vi "Actor Core.vi"(8 "error in":errorcluster, 11 "Nested in":refnum<class "Productos.lvclass">) -> (0 "error out":errorcluster, 3 "Actor out":refnum<class "Actor.lvclass">)   [LabVIEW 2020, in "Productos.lvlib" / "Productos.lvclass"]
doc: "(<B>Filename</B>: Actor Framework.lvlib:Actor.lvclass:Actor Core.vi)\n\nReceives messages to the actor, reacts to them, and initiates any error handling that may shut the actor down.\n\nDescendant classes may override this VI to append parallel tasks for the actor to complete while it handles messages. Overrides use the Call Parent Method node."
uses:
  Productos.lvclass
  <vilib>/ActorFramework/Actor/Actor.lvclass
  <vilib>/ActorFramework/Stop Msg/Stop Msg.lvclass
  Productos Messages/Producto extraccion Msg/Producto extraccion Msg.lvclass
  Productos Messages/Inventory Msg/Inventory Msg.lvclass
  Productos Messages/Cobro Prod Msg/Cobro Prod Msg.lvclass
panel:
  in  "Cancel Button":bool
  in  "Inventario":bool
  in  "Listo":bool
  out "Total":dbl format="$ %#_6f"
  in  "Chicles":bool
  in  "Cacahuates":bool
  in  "Galletas":bool
  in  "Chocolate":bool
  in  "Sabritas":bool
  in  "Doritos":bool
  in  "Pepsi":bool
  in  "Coca":bool
  out "Productos":T1
  # "Para realizar su pedido haga click en el boton de lo que vaya a ordenar"
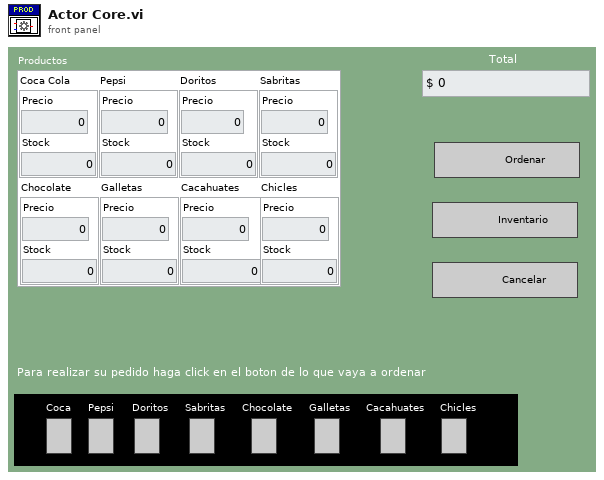
[diagram p1: front panel]
types:
  T1 = cluster{"Coca Cola":cluster{"Precio":dbl, "Stock":dbl}, "Pepsi":cluster{"Precio":dbl, "Stock":dbl}, "Doritos":cluster{"Precio":dbl, "Stock":dbl}, "Sabritas":cluster{"Precio":dbl, "Stock":dbl}, "Chocolate":cluster{"Precio":dbl, "Stock":dbl}, "Galletas":cluster{"Precio":dbl, "Stock":dbl}, "Cacahuates":cluster{"Precio":dbl, "Stock":dbl}, "Chicles":cluster{"Precio":dbl, "Stock":dbl}}
  T2 = cluster{"Stop":refnum<user-event>, "Total":refnum<user-event>, "Productos":refnum<user-event>}
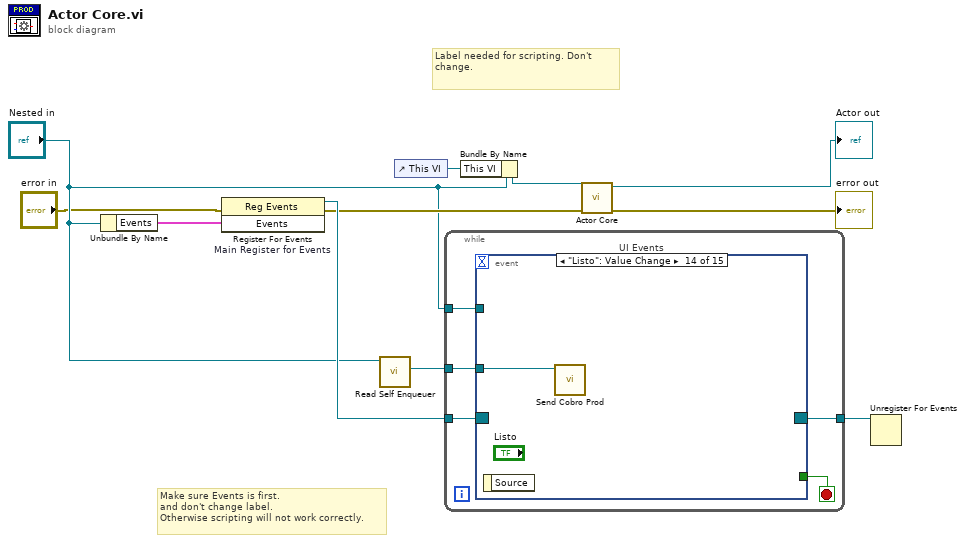
[diagram p0: block diagram]
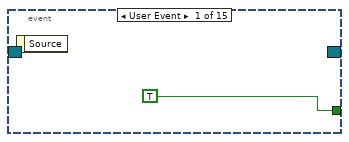
[diagram p2: hidden frame]
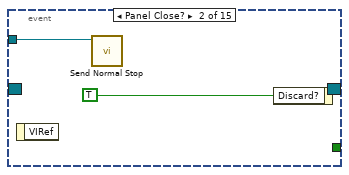
[diagram p3: hidden frame]
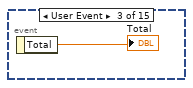
[diagram p4: hidden frame]
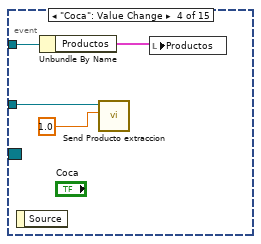
[diagram p5: hidden frame]
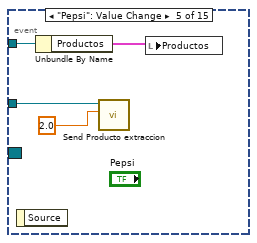
[diagram p6: hidden frame]
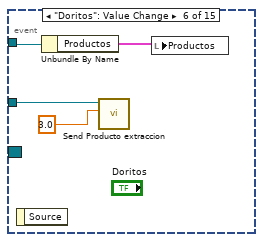
[diagram p7: hidden frame]
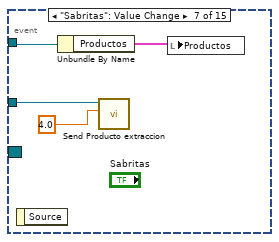
[diagram p8: hidden frame]
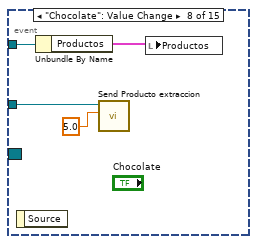
[diagram p9: hidden frame]
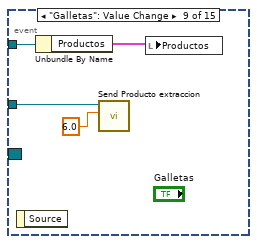
[diagram p10: hidden frame]
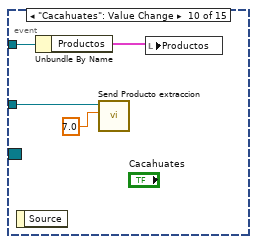
[diagram p11: hidden frame]
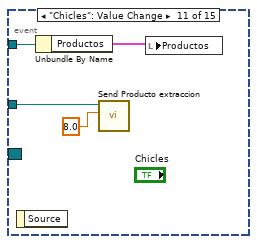
[diagram p12: hidden frame]
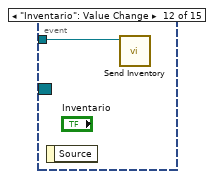
[diagram p13: hidden frame]
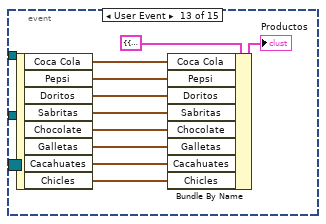
[diagram p14: hidden frame]
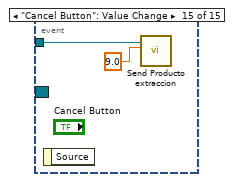
[diagram p15: hidden frame]
diagram:
  # "Label needed for scripting. Don't change."
  # "Make sure Events is first.\nand don't change label.\nOtherwise scripting will not work correctly."
  n1 = Unbundle By Name("Nested in") -> ("Events"=w8:T2)
  n2 = register-events "Main Register for Events"(error in="error in", w8) -> (reference out=w9:refnum<event-registration>, error out=w5:errorcluster)  [unwired: 1 in]
  n3 = call <vilib>:"Read Self Enqueuer.vi"("Actor"="Nested in") -> ("Self Enqueuer"=w6:refnum<class "Message Enqueuer.lvclass">)  [unwired: 10 in]
  n4 = control-ref of="This VI"() -> (w3:refnum<vi>)
  n5 = while {
    tunnel: w9 -> [w16]
    tunnel: [w14] -> w7
    tunnel: w6 -> [w13]
    tunnel: "Nested in" -> [w12]
    stop <- w15 stop-if-true
    n6 = event "UI Events" shown="[13] \"Listo\": Value Change" {
      selector: w16 -> [_ _ _ _ _ _ _ _ _ _ _ _ _ _ _]
      dyn-events: [_ _ _ _ _ _ _ _ _ _ _ _ _ _ _] -> w14
      timeout: _ -> [_ _ _ _ _ _ _ _ _ _ _ _ _ _ _]
      tunnel: [TRUE _ _ _ _ _ _ _ _ _ _ _ _ _ _] -> w15
      tunnel: w13 -> [_ w18 _ w24 w28 w32 w36 w40 w44 w48 w52 w53 _ w64 w65]
      tunnel: w12 -> [_ _ _ w21 w25 w29 w33 w38 w42 w46 w50 _ _ _ _]
      event User Event {
        n7 = event-data() -> ()  [unwired: 1 in, 1 out]
      }
      event Panel Close? {
        n8 = event-data() -> ()  [unwired: 1 in, 1 out]
        n9 = call <vilib>:"Send Normal Stop.vi"("Message Enqueuer"=w18) -> ()  [unwired: 10 in, 1 out]
        n10 = event-data("Discard?"=TRUE) -> ()  [unwired: 1 in, 1 out]
      }
      event User Event {
        n11 = event-data() -> ("Total"=→"Total":dbl)  [unwired: 1 in]
      }
      event "Coca": Value Change {
        n12 = event-data() -> ()  [unwired: 1 in, 1 out]
        n13 = Unbundle By Name(w21) -> ("Productos"=w22:T1)
        n14 = call "Send Producto extraccion.vi"("Indicador"=1.0, "Message Enqueuer"=w24) -> ()  [unwired: 8 in, 2 out]
        n15 = local write "Productos"(w22) -> ()
      }
      event "Pepsi": Value Change {
        n16 = event-data() -> ()  [unwired: 1 in, 1 out]
        n17 = Unbundle By Name(w25) -> ("Productos"=w26:T1)
        n18 = call "Send Producto extraccion.vi"("Indicador"=2.0, "Message Enqueuer"=w28) -> ()  [unwired: 8 in, 2 out]
        n19 = local write "Productos"(w26) -> ()
      }
      event "Doritos": Value Change {
        n20 = event-data() -> ()  [unwired: 1 in, 1 out]
        n21 = Unbundle By Name(w29) -> ("Productos"=w30:T1)
        n22 = call "Send Producto extraccion.vi"("Indicador"=3.0, "Message Enqueuer"=w32) -> ()  [unwired: 8 in, 2 out]
        n23 = local write "Productos"(w30) -> ()
      }
      event "Sabritas": Value Change {
        n24 = event-data() -> ()  [unwired: 1 in, 1 out]
        n25 = Unbundle By Name(w33) -> ("Productos"=w34:T1)
        n26 = call "Send Producto extraccion.vi"("Indicador"=4.0, "Message Enqueuer"=w36) -> ()  [unwired: 8 in, 2 out]
        n27 = local write "Productos"(w34) -> ()
      }
      event "Chocolate": Value Change {
        n28 = event-data() -> ()  [unwired: 1 in, 1 out]
        n29 = Unbundle By Name(w38) -> ("Productos"=w37:T1)
        n30 = call "Send Producto extraccion.vi"("Indicador"=5.0, "Message Enqueuer"=w40) -> ()  [unwired: 8 in, 2 out]
        n31 = local write "Productos"(w37) -> ()
      }
      event "Galletas": Value Change {
        n32 = event-data() -> ()  [unwired: 1 in, 1 out]
        n33 = Unbundle By Name(w42) -> ("Productos"=w41:T1)
        n34 = call "Send Producto extraccion.vi"("Indicador"=6.0, "Message Enqueuer"=w44) -> ()  [unwired: 8 in, 2 out]
        n35 = local write "Productos"(w41) -> ()
      }
      event "Cacahuates": Value Change {
        n36 = event-data() -> ()  [unwired: 1 in, 1 out]
        n37 = Unbundle By Name(w46) -> ("Productos"=w45:T1)
        n38 = call "Send Producto extraccion.vi"("Indicador"=7.0, "Message Enqueuer"=w48) -> ()  [unwired: 8 in, 2 out]
        n39 = local write "Productos"(w45) -> ()
      }
      event "Chicles": Value Change {
        n40 = event-data() -> ()  [unwired: 1 in, 1 out]
        n41 = Unbundle By Name(w50) -> ("Productos"=w49:T1)
        n42 = call "Send Producto extraccion.vi"("Indicador"=8.0, "Message Enqueuer"=w52) -> ()  [unwired: 8 in, 2 out]
        n43 = local write "Productos"(w49) -> ()
      }
      event "Inventario": Value Change {
        n44 = event-data() -> ()  [unwired: 1 in, 1 out]
        n45 = call "Send Inventory.vi"("Message Enqueuer"=w53) -> ()  [unwired: 9 in, 2 out]
      }
      event User Event {
        n46 = event-data() -> ("Coca Cola"=w61:cluster{"Precio":dbl, "Stock":dbl}, "Pepsi"=w60:cluster{"Precio":dbl, "Stock":dbl}, "Doritos"=w59:cluster{"Precio":dbl, "Stock":dbl}, "Sabritas"=w58:cluster{"Precio":dbl, "Stock":dbl}, "Chocolate"=w57:cluster{"Precio":dbl, "Stock":dbl}, "Galletas"=w56:cluster{"Precio":dbl, "Stock":dbl}, "Cacahuates"=w55:cluster{"Precio":dbl, "Stock":dbl}, "Chicles"=w54:cluster{"Precio":dbl, "Stock":dbl})  [unwired: 1 in]
        n47 = Bundle By Name(cluster=T1 {"Coca Cola"={"Precio"=0.0, "Stock"=0.0}, "Pepsi"={"Precio"=0.0, "Stock"=0.0}, "Doritos"={"Precio"=0.0, "Stock"=0.0}, "Sabritas"={"Precio"=0.0, "Stock"=0.0}, "Chocolate"={"Precio"=0.0, "Stock"=0.0}, "Galletas"={"Precio"=0.0, "Stock"=0.0}, "Cacahuates"={"Precio"=0.0, "Stock"=0.0}, "Chicles"={"Precio"=0.0, "Stock"=0.0}} ("Productos"), "Coca Cola"=w61, "Pepsi"=w60, "Doritos"=w59, "Sabritas"=w58, "Chocolate"=w57, "Galletas"=w56, "Cacahuates"=w55, "Chicles"=w54) -> (→"Productos":T1)
      }
      event "Listo": Value Change {
        n48 = event-data() -> ()  [unwired: 1 in, 1 out]
        n49 = call "Send Cobro Prod.vi"("Message Enqueuer"=w64) -> ()  [unwired: 9 in, 2 out]
      }
      event "Cancel Button": Value Change {
        n50 = event-data() -> ()  [unwired: 1 in, 1 out]
        n51 = call "Send Producto extraccion.vi"("Indicador"=9.0, "Message Enqueuer"=w65) -> ()  [unwired: 8 in, 2 out]
      }
    }
  }
  n52 = Bundle By Name(cluster="Nested in", "This VI"=w3) -> (w4:refnum<class "Productos.lvclass">)
  n53 = call-parent "Actor Core.vi"("error in"=w5, "Actor in"=w4) -> ("error out"=→"error out":errorcluster, "Actor out"=→"Actor out":refnum<class "Actor.lvclass">)  [unwired: 8 in]
  n54 = Unregister For Events(event registration refnum=w7) -> ()  [unwired: 1 in, 1 out]
